vi "L0_Init_ASICtest.vi"(8 "error in":errorcluster, 11 "connection ID in":refnum<k5>) -> (0 "error out":errorcluster, 3 "connection ID out":refnum<k5>)   [LabVIEW 2012]
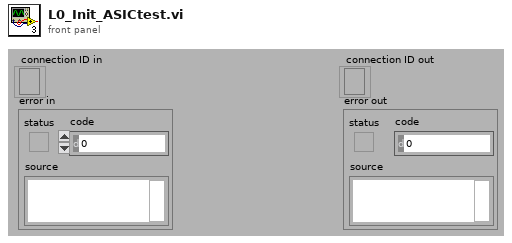
[diagram p1: front panel]
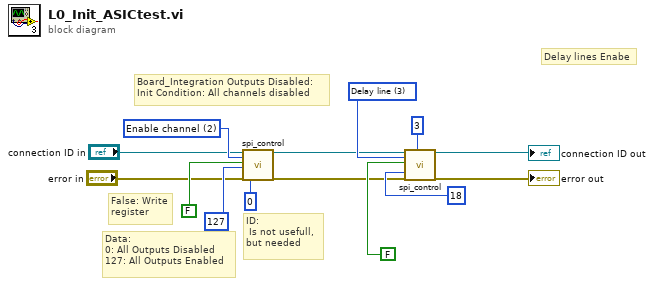
[diagram p0: block diagram]
diagram:
  w5 = u16 3 items=["Attenuation", "Clipping", "Enable channel", "Delay line", "ASIC"] ("Device")
  w13 = u16 2 items=["Attenuation", "Clipping", "Enable channel", "Delay line", "ASIC"] ("Device")
  # "False: Write\nregister"
  # "Data:\n0: All Outputs Disabled\n127: All Outputs Enabled"
  # "ID:\n Is not usefull, \nbut needed"
  # "Board_Integration Outputs Disabled:\nInit Condition: All channels disabled"
  # "Delay lines Enabe"
  n1 = call "spi_control.vi"("connection ID"="connection ID in", "Device"=w13, "Read/#write"=FALSE, "Data"=127, "error in"="error in", "Id in"=0) -> ("connection ID out"=w2:refnum<k5>, "error out 2"=w1:errorcluster)  [unwired: 6 in, 6 out]
  n2 = call "spi_control.vi"("connection ID"=w2, "Device"=w5, "Read/#write"=FALSE, "Register or channel"=18, "error in"=w1, "chip delay"=3) -> ("connection ID out"=→"connection ID out":refnum<k5>, "error out 2"=→"error out":errorcluster)  [unwired: 6 in, 6 out]
